vi "Configure Level Trigger_20220926.vi"(0 "device session in":refnum<class "Device Session.lvclass">, 7 "trigger level hi (V)":dbl, 9 "trigger level lo (V)":dbl, 11 "error in":errorcluster) -> (4 "device session out":refnum<class "Device Session.lvclass">, 15 "error out":errorcluster)   [LabVIEW 2021, in "Device Session.lvclass"]
doc: "Configures the level trigger for a channel. You can specify the trigger slope, the trigger level, and whether the device should trigger on an input below or above the specified trigger level. You must run the <B>Configure Channel</B> VI before running this VI.\n\n<B>Input Parameters</B>\n\n<B>device session in</B> is a reference to the Device Session object, which contains a session to each instrument design library used in this sample project. This parameter is obtained from the 'Open Session' VI.\n\n<B>trigger source</B> specifies the channel to monitor for trigger conditions.\n\n<B>trigger when</B> specifies whether the device should trigger if the input is below or above the specified 'level'.\n\n<B>trigger level (V)</B> specifies the voltage threshold for the trigger.\n\n<B>instance</B> specifies either instance A or B of the trigger to use.\n\n<B>error in</B> describes error conditions that occur before this node runs. This input provides standard 'error in' functionality.\n\n<B>Output Parameters</B>\n\n<B>device session out</B> passes a reference to the session to the next VI.\n\n<B>error out</B> contains error information. This output provides standard 'error out' functionality."
uses:
  Device Session.lvclass
  Device Session.lvclass/Device Session.ctl
  <instrlib>/_niInstr/Data Trigger/v1/Shared/Public/Level Configuration FXP(+-,18,1).ctl
  <instrlib>/_niInstr/Data Trigger/v1/Shared/Public/Level Configuration Trigger When.ctl
  <vilib>/Utility/error.llb/Error Cluster From Error Code.vi
  <vilib>/rvi/errors/niLvFpgaAdjustHostInterfaceError.vi
  <vilib>/rvi/interface/nirviReadWriteControl/nirviReadWriteControl.xnode
  FPGA Refnum.ctl
  <vilib>/rvi/interface/Simulation/niFpgaSimulationCallBeginRW.vi
  <instrlib>/_niInstr/Data Trigger/v1/Shared/niInstr Data Trigger v1 Shared.lvlib
  NiFpgaLv.dll
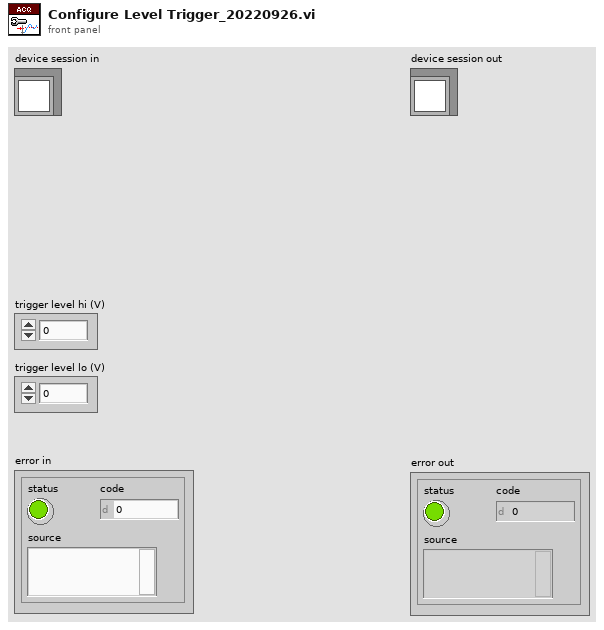
[diagram p1: front panel]
types:
  T1 = typedef "niInstr Data Trigger v1 Shared.lvlib/Level Configuration Trigger When.ctl" = enum8{"Trigger Above", "Trigger Below"}
  T2 = typedef "niInstr Data Trigger v1 Shared.lvlib/Level Configuration FXP(+-,18,1).ctl" = cluster{"level":fxp<+/-,18,1>, "trigger when":T1}
  T3 = enum16{"Immediate", "A", "B", "OR", "AND", "A THEN B", "B THEN A", "High Resolution"}
  T4 = typedef "Device Session.lvclass/Device Session Object.ctl" = cluster{"fpga reference":T5, "reg bus":refnum<class "niInstr FIFO Register Bus v1 Host.lvclass">, "subsystem map":refnum<class "niInstr Subsystem Map v1 Host.lvclass">, "cal data":refnum<class "niHSAI Cal Data v1 Host.lvclass">, "config":refnum<class "niHSAI Group A Config v1 Host.lvclass">, "acquisition":refnum<class "niInstr Multirecord Acquisition v1 Host.lvclass">, "number of selected acq channels":u8, "selected acq channels":bool[], "number of channels":u32, "configured channels":bool[], "acq configuration":cluster{"number of samples":u64, "number of records":u64, "pretrigger samples":u64}, "actual channel configuration":T6[], "sample clock rate (Hz)":dbl, "scaling coefficients":T10[]}
  T5 = typedef "Device Session.lvclass/FPGA Refnum.ctl" = refnum<k20>
  T6 = typedef "niHSAI Types v1 Host.lvlib/Channel Configuration.ctl" = cluster{"channel":u32, "coupling":T7, "impedance":T8, "bandwidth":T9, "vertical range":dbl, "vertical offset":dbl}
  T7 = typedef "niHSAI Types v1 Host.lvlib/Coupling.ctl" = enum8{"Default", "DC", "AC"}
  T8 = typedef "niHSAI Types v1 Host.lvlib/Impedance.ctl" = enum8{"Default", "1 mega ohm", "50 ohm"}
  T9 = typedef "niHSAI Types v1 Host.lvlib/Bandwidth.ctl" = enum8{"Default", "Full Bandwidth", "Anti-alias Filter", "150 MHz"}
  T10 = typedef "niInstr Multirecord Acquisition v1 Host.lvclass/Scaling Coefficient.ctl" = cluster{"gain":dbl, "offset":dbl}
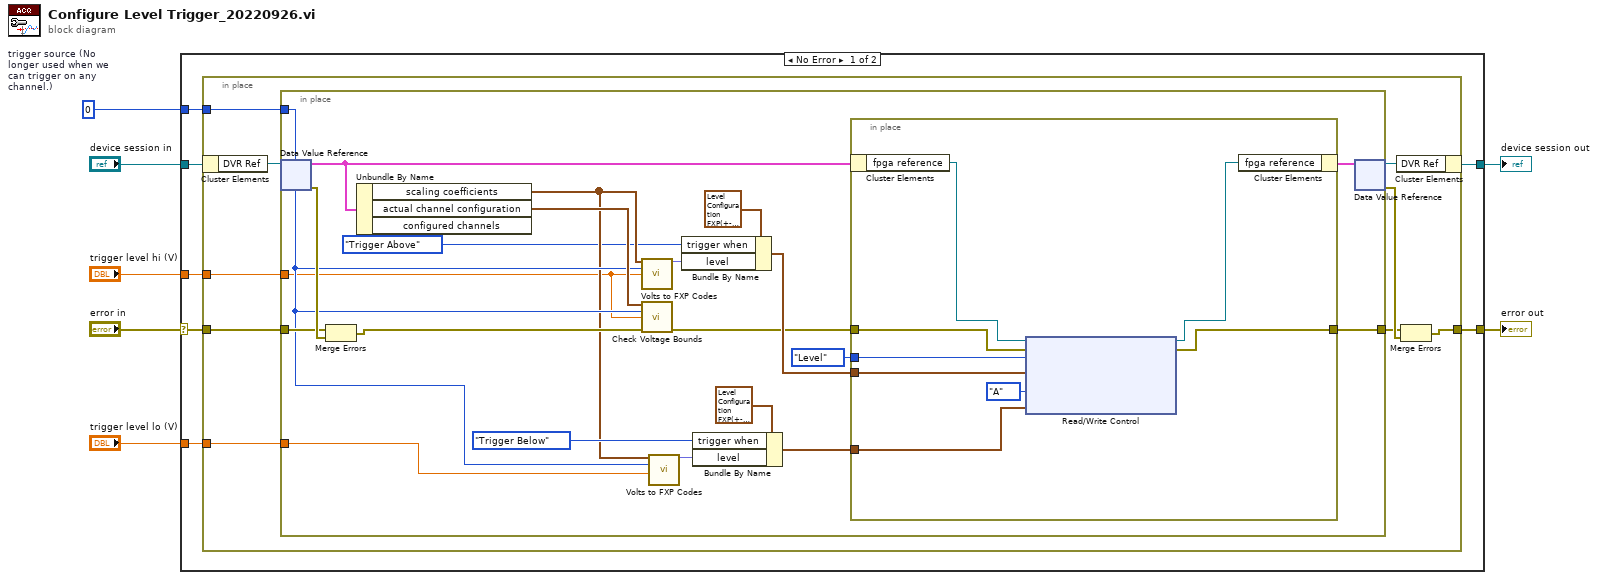
[diagram p0: block diagram]
diagram:
  w3 = u8 0  # trigger source (No longer used when we can trigger on any channel.)
  n1 = case shown="No Error" "error in" {
    selector: "error in" -> [w14 w54]
    tunnel: "device session in" -> [w10 w53]
    tunnel: [w9 w53] -> w6
    tunnel: [w11 w54] -> w7
    tunnel: w3 -> [w13 _]
    tunnel: "trigger level hi (V)" -> [w12 _]
    tunnel: "trigger level lo (V)" -> [w8 _]
    frame No Error {
      n2 = in-place {
        in-place-border: w14 -> [w23]
        in-place-border: w13 -> [w22]
        in-place-border: w12 -> [w19]
        in-place-border: [w18] -> w11
        in-place-border: w8 -> [w15]
        n3 = in-place-cluster #1(w10) -> ("DVR Ref"=w17:refnum<data-value>)
        n4 = in-place {
          in-place-border: w23 -> [w43]
          in-place-border: w22 -> [w29]
          in-place-border: [w41] -> w20
          in-place-border: w19 -> [w27]
          in-place-border: w15 -> [w25]
          n5 = in-place-dvr #2(w17) -> (w36:T4, w44:errorcluster)
          n6 = Merge Errors(w43, w44) -> (w34:errorcluster)
          n7 = Unbundle By Name(w36) -> ("scaling coefficients"=w28:T10[], "actual channel configuration"=w33:T6[])  [unwired: 1 out]
          n8 = call "Volts to FXP Codes.vi"("scaling coefficients"=w28, "channel index"=w29, "level (V)"=w27) -> ("codes"=w38:fxp<+/-,18,1>)  [unwired: 12 in]
          n9 = call "Check Voltage Bounds.vi"("channel configuration"=w33, "trigger source"=w29, "level (V)"=w27, "error in"=w34) -> ("error out"=w37:errorcluster)  [unwired: 11 in]
          n10 = call "Volts to FXP Codes.vi"("scaling coefficients"=w28, "channel index"=w29, "level (V)"=w25) -> ("codes"=w30:fxp<+/-,18,1>)  [unwired: 12 in]
          n11 = Bundle By Name(cluster=T2 {"level"=0.0, "trigger when"=enum."Trigger Above"} ("configuration"), "trigger when"=Level_Configuration_Trigger_When."Trigger Above", "level"=w38) -> (w40:T2)
          n12 = Bundle By Name(cluster=T2 {"level"=0.0, "trigger when"=enum."Trigger Above"} ("configuration"), "trigger when"=Level_Configuration_Trigger_When."Trigger Below", "level"=w30) -> (w26:T2)
          n13 = in-place {
            in-place-border: enum16{"Edge", "Level", "Custom"}."Level" ("trigger.select 0") -> [w52]
            in-place-border: [w51] -> w41
            in-place-border: w40 -> [w50]
            in-place-border: w37 -> [w49]
            in-place-border: w26 -> [w46]
            n14 = in-place-cluster #3(w36) -> ("fpga reference"=w47:T5)
            n15 = xnode "Read/Write Control"("FPGA VI Reference In"=w47, "error in"=w49, "trigger.type A"=w52, "trigger.level A"=w50, "trigger.combination type"=T3."A" ("trigger.combination.type"), "trigger.level B"=w46) -> ("FPGA VI Reference Out"=w48:T5, "error out"=w51:errorcluster)
            n16 = in-place-cluster #3("fpga reference"=w48) -> (w35:T4)
          }
          n17 = in-place-dvr #2(w35) -> (w16:refnum<data-value>, w21:errorcluster)
        }
        n18 = in-place-cluster #1("DVR Ref"=w16) -> (w9:refnum<class "Device Session.lvclass">)
        n19 = Merge Errors(w20, w21) -> (w18:errorcluster)
      }
    }
    frame Error {
    }
  }
  "error out" <- w7
  "device session out" <- w6
